vi "Read Response.vi"(7 "Timeout (s)":dbl, 8 "error in (no error)":errorcluster, 10 "regular expression":string, 11 "PN532 COM Port":refnum<visa-resource-name>) -> (0 "error out":errorcluster, 1 "Response Data":string, 2 "Found?":bool, 3 "PN532 COM Port Out":refnum<visa-resource-name>)   [LabVIEW 2012, in "NFC Driver.lvlib"]
doc: "Reads from the serial port specified by \"PN532 COM Port\" until a match for the regular expression specified by \"Regular Expression\" is found or until time equal or greater to that specified by \"Timeout (s)\" has elapsed.\n\n\"Response Data\" will return any information found after the matched regular expression.\n\nThe execution of this VI is also interrupted if an error occurs."
uses:
  NFC Driver.lvlib
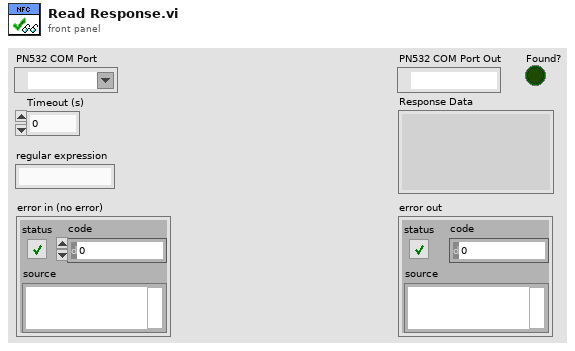
[diagram p1: front panel]
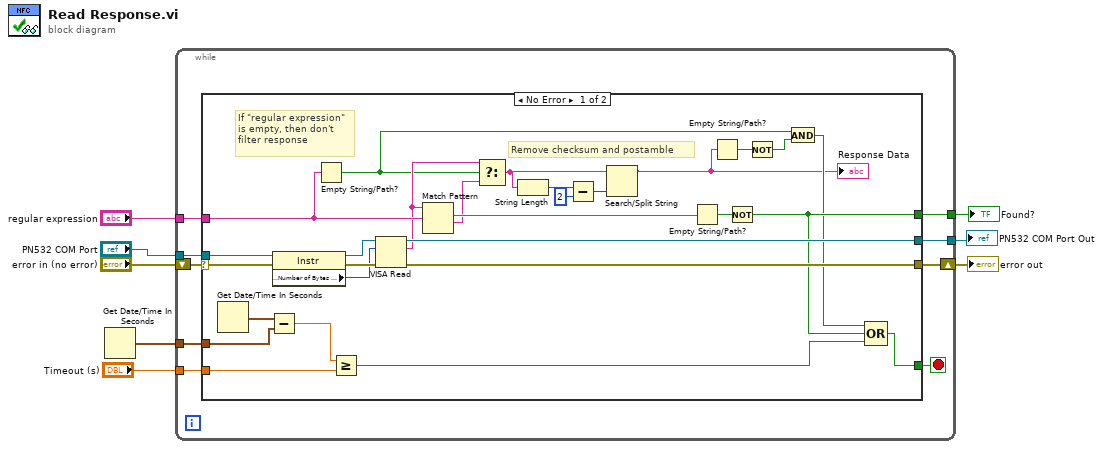
[diagram p0: block diagram]
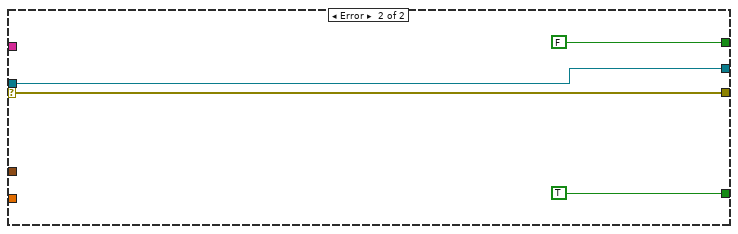
[diagram p2: hidden frame]
diagram:
  n1 = Get Date/Time In Seconds() -> (seconds since 1Jan1904=w2:timestamp)
  n2 = while {
    tunnel: "PN532 COM Port" -> [w17]
    tunnel: "regular expression" -> [w16]
    tunnel: [w15] -> w5
    tunnel: [w14] -> w4
    shift-right: [w13] -> w3
    shift-left: "error in (no error)" -> [w12]
    tunnel: w2 -> [w10]
    tunnel: "Timeout (s)" -> [w9]
    stop <- w11 stop-if-true
    n3 = case shown="No Error" w12 {
      selector: w12 -> [w37 w46]
      tunnel: w17 -> [w40 w47]
      tunnel: w16 -> [w29 _]
      tunnel: [w39 w47] -> w15
      tunnel: [w30 FALSE] -> w14
      tunnel: [w38 w46] -> w13
      tunnel: [w31 TRUE] -> w11
      tunnel: w10 -> [w35 _]
      tunnel: w9 -> [w33 _]
      frame No Error {
        # "Remove checksum and postamble"
        # "If \"regular expression\"\nis empty, then don't \nfilter response"
        n4 = Get Date/Time In Seconds() -> (seconds since 1Jan1904=w36:timestamp)
        n5 = Subtract(x=w36, y=w35) -> (x-y=w34:dbl)
        n6 = property class="Instr"(reference=w40, error in=w37) -> (reference out=w43:refnum<visa-resource-name>, error out=w45:errorcluster, "Serial Settings:Number of Bytes at Serial Port"=w44:u32)
        n7 = Empty String/Path?(string/path=w29) -> (empty?=w25:bool)
        n8 = Greater Or Equal?(x=w34, y=w33) -> (x >= y?=w32:bool)
        n9 = VISA Read(VISA resource name=w43, byte count=w44, error in (no error)=w45) -> (VISA resource name out=w39:refnum<visa-resource-name>, read buffer=w27:string, error out=w38:errorcluster)  [unwired: 1 out]
        n10 = Match Pattern(string=w27, regular expression=w29) -> (match substring=w42:string, after substring=w28:string)  [unwired: 1 in, 2 out]
        n11 = Select(t=w27, s=w25, f=w28) -> (s? t:f=w20:string)
        n12 = String Length(string=w20) -> (length=w22:i32)
        n13 = Subtract(x=w22, y=2) -> (x-y=w19:i32)
        n14 = Search/Split String(string=w20, offset (0)=w19) -> (substring before match=w18:string)  [unwired: 1 in, 2 out]
        "Response Data" <- w18
        n15 = Empty String/Path?(string/path=w42) -> (empty?=w41:bool)
        n16 = Empty String/Path?(string/path=w18) -> (empty?=w26:bool)
        n17 = Not(x=w41) -> (.not. x?=w30:bool)
        n18 = Not(x=w26) -> (.not. x?=w23:bool)
        n19 = And(x=w25, y=w23) -> (x .and. y?=w24:bool)
        n20 = Compound Arithmetic op=OR(w24, w30, w32) -> (w31:bool)
      }
      frame Error {
      }
    }
  }
  "PN532 COM Port Out" <- w5
  "Found?" <- w4
  "error out" <- w3
